vi "SwerveDriveSetOutputs.vi"(9 "VelocitySetpoints":dbl[](array[numeric]), 11 "AngleSetpoints":dbl[](array[numeric])) -> ()   [LabVIEW 2020]
uses:
  Robot Global Data.vi
panel:
  # "Copied and pasted from EF's code. not complex and honestly not really needed but if it\nmakes him happy then it is worth having"
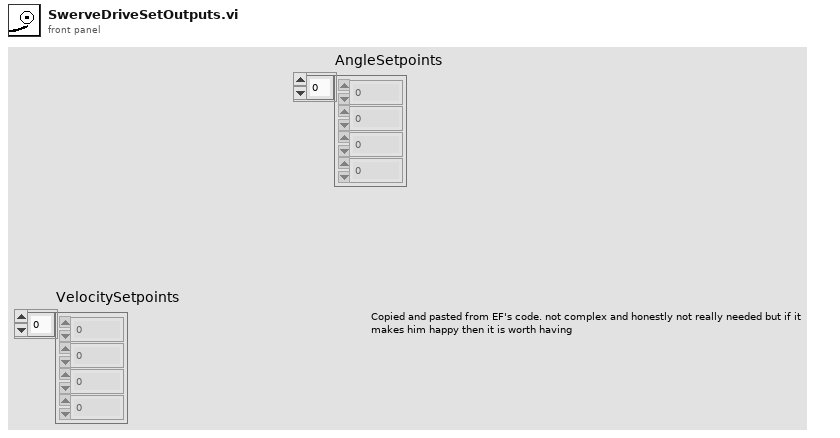
[diagram p1: front panel]
types:
  T1 = typedef "WPI_MotorControlDeviceRef.ctl" = cluster{"DeviceStatus":errorcluster, "Type":T2, "PWM":cluster{"PWM Channel":T3, "DeadBand":T4}, "CAN":cluster{"Device Number":u8, "SetOutput VI Ref":variant, "GetOutput VI Ref":variant, "Enable VI Ref":variant, "Disable VI Ref":variant, "Data":variant}, "Invert":bool, "DIO PWM":cluster{"PWM \"Enable\" Channel":T3, "DIOChannel":T5, "PWM Rate":dbl}}
  T2 = typedef "WPI_MotorControlType.ctl" = enum16{"PWM", "CAN", "DIO PWM"}
  T3 = typedef "FPGA_DIOPWMChannel.ctl" = enum8{"PWM 0", "PWM 1", "PWM 2", "PWM 3", "PWM 4", "PWM 5", "PWM 6", "PWM 7", "PWM 8", "PWM 9", "PWM MXP 0", "PWM MXP 1", "PWM MXP 2", "PWM MXP 3", "PWM MXP 4", "PWM MXP 5", "PWM MXP 6", "PWM MXP 7", "PWM MXP 8", "PWM MXP 9", "Invalid"}
  T4 = typedef "WPI_PWMDeadband.ctl" = cluster{"Name":string, "maxPositivePwm":i32, "minPositivePwm":i32, "centerPwm":i32, "maxNegativePwm":i32, "minNegativePwm":i32, "angularRange":u16}
  T5 = typedef "FPGA_DIOChannel.ctl" = enum8{"DIO 0", "DIO 1", "DIO 2", "DIO 3", "DIO 4", "DIO 5", "DIO 6", "DIO 7", "DIO 8", "DIO 9", "DIO MXP 0", "DIO MXP 1", "DIO MXP 2", "DIO MXP 3", "DIO MXP 4", "DIO MXP 5", "DIO MXP 6", "DIO MXP 7", "DIO MXP 8", "DIO MXP 9", "DIO MXP 10", "DIO MXP 11", "DIO MXP 12", "DIO MXP 13", "DIO MXP 14", "DIO MXP 15", "SPI Port CS1", "SPI Port CS2", "SPI Port CS3", "SPI Port MISO", "SPI Port MOSI", "Invalid"}
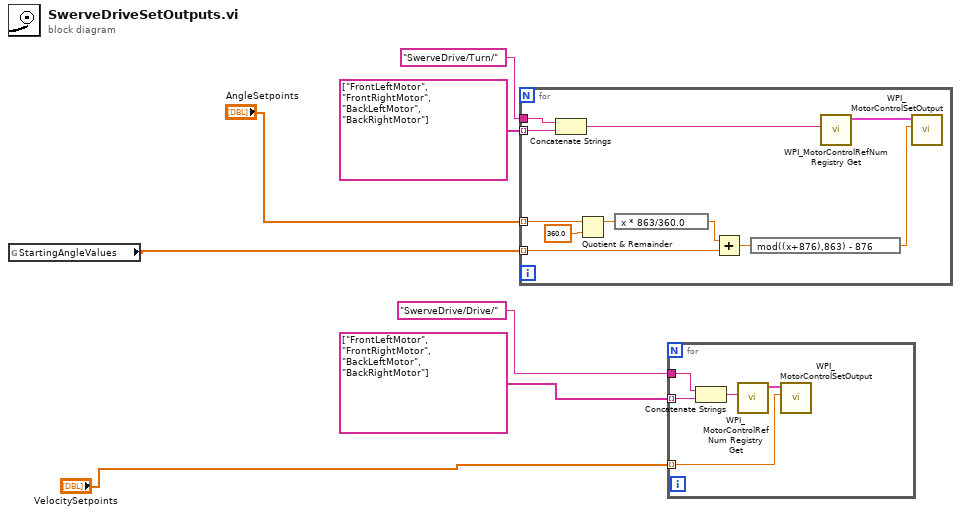
[diagram p0: block diagram]
diagram:
  n1 = global read "Robot Global Data.vi" "StartingAngleValues"() -> (w1:dbl[])
  n2 = for {
    tunnel: "AngleSetpoints" -> [w9] mode=indexing
    tunnel: string[] ["FrontLeftMotor", "FrontRightMotor", "BackLeftMotor", "BackRightMotor"] -> [w16] mode=indexing
    tunnel: "SwerveDrive/Turn/" ("refnum name") -> [w17]
    tunnel: w1 -> [w8] mode=indexing
    n3 = Concatenate Strings(w17, w16) -> (w15:string)
    n4 = Quotient & Remainder(x=w9, y=360.0) -> (x-y*floor(x/y)=w12:dbl)  [unwired: 1 out]
    n5 = expression code="x * 863/360.0"(w12) -> (w10:dbl)
    n6 = Add(x=w10, y=w8) -> (x+y=w14:dbl)
    n7 = expression code="mod((x+876),863) - 876"(w14) -> (w11:dbl)
    n8 = call <vilib>:"WPI_MotorControlRefNum Registry Get.vi"("refnum name"=w15) -> ("MotorControlDevRef"=w18:T1)  [unwired: 9 in, 1 out]
    n9 = call <vilib>:"WPI_MotorControlSetOutput.vi"("Output"=w11, "MotorControlDevRef"=w18) -> ()  [unwired: 7 in, 3 out]
  }
  n10 = for {
    tunnel: string[] ["FrontLeftMotor", "FrontRightMotor", "BackLeftMotor", "BackRightMotor"] -> [w21] mode=indexing
    tunnel: "SwerveDrive/Drive/" ("refnum name") -> [w22]
    tunnel: "VelocitySetpoints" -> [w19] mode=indexing
    n11 = Concatenate Strings(w22, w21) -> (w20:string)
    n12 = call <vilib>:"WPI_MotorControlRefNum Registry Get.vi"("refnum name"=w20) -> ("MotorControlDevRef"=w23:T1)  [unwired: 9 in, 1 out]
    n13 = call <vilib>:"WPI_MotorControlSetOutput.vi"("Output"=w19, "MotorControlDevRef"=w23) -> ()  [unwired: 7 in, 3 out]
  }
